vi "Pass Fail Result to Color.vi"(11 "Pass?":bool) -> (3 "Color Value":u32)   [LabVIEW 2014]
uses:
  Globals/Pass Fail Result Colors.vi
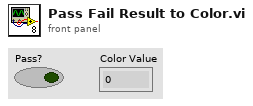
[diagram p1: front panel]
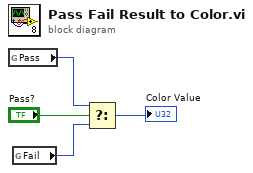
[diagram p0: block diagram]
diagram:
  n1 = global read "Pass Fail Result Colors.vi" "Pass"() -> (w1:u32)
  n2 = global read "Pass Fail Result Colors.vi" "Fail"() -> (w2:u32)
  n3 = Select(t=w1, s="Pass?", f=w2) -> (s? t:f=→"Color Value":u32)
